vi "Read Inputs from system.vi"(8 "error in":errorcluster, 11 "ExampleStateMachine runtime in":refnum<class "ExampleStateMachine runtime.lvclass">) -> (0 "error out":errorcluster, 2 "Inputs from system":T1, 3 "ExampleStateMachine runtime out":refnum<class "ExampleStateMachine runtime.lvclass">)   [LabVIEW 2017, in "ExampleStateMachine runtime.lvclass"]
uses:
  ExampleStateMachine runtime.lvclass
  configuration/input data indices.ctl
  ExampleStateMachine runtime.lvclass/ExampleStateMachine runtime.ctl
  configuration/ExampleStateMachine configuration.lvclass
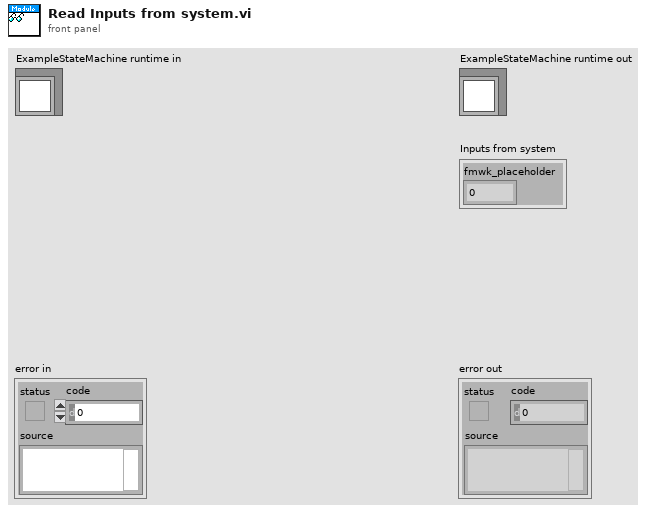
[diagram p1: front panel]
types:
  T1 = typedef "ExampleStateMachine configuration.lvclass/input data indices.ctl" = cluster{"fmwk_placeholder":i32}
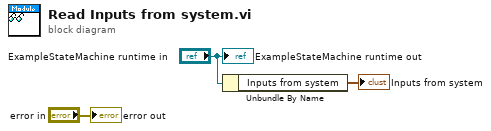
[diagram p0: block diagram]
diagram:
  n1 = Unbundle By Name("ExampleStateMachine runtime in") -> ("Inputs from system"=→"Inputs from system":T1)
  "error out" <- "error in"
  "ExampleStateMachine runtime out" <- "ExampleStateMachine runtime in"
